vi "config.vi"(8 "error in (no error)":errorcluster, 10 "Configuration":T2={"Config Dir"=path "/home/ttsai/Documents/stash/ts_tcs_ofc/configData", "Config File Name"="optiPSSN_x00.ctrl", "Inst Name"=enum."lsst", "State 0 File Name"="state0inDof.txt", "Weighting File Name"="imgQualWgt.txt", "PSSN Alpha File Name"="pssn_alpha.txt", "Authority Files"={"Rigid Body Stroke File"="rbStroke.txt", "M1M3 Subsystem"={"Mirror"="M1M3", "Actuatro Force File"="M1M3_1um_156_force.DAT"}, "M2 Subsystem"={"Mirror"="M2", "Actuatro Force File"="M2_1um_force.DAT"}, "Num of Bending Mode"=20}}, 11 "OptCtrl in":refnum<class "OptCtrl.lvclass">) -> (0 "error out":errorcluster, 3 "OptCtrl out":refnum<class "OptCtrl.lvclass">)   [LabVIEW 2016, in "OptCtrl.lvclass"]
doc: "Do the configuration of optimal comtrol (OC)."
uses:
  OptCtrl.lvclass
  StrictDef/InstName.ctl
  OptCtrl.lvclass/OptCtrl.ctl
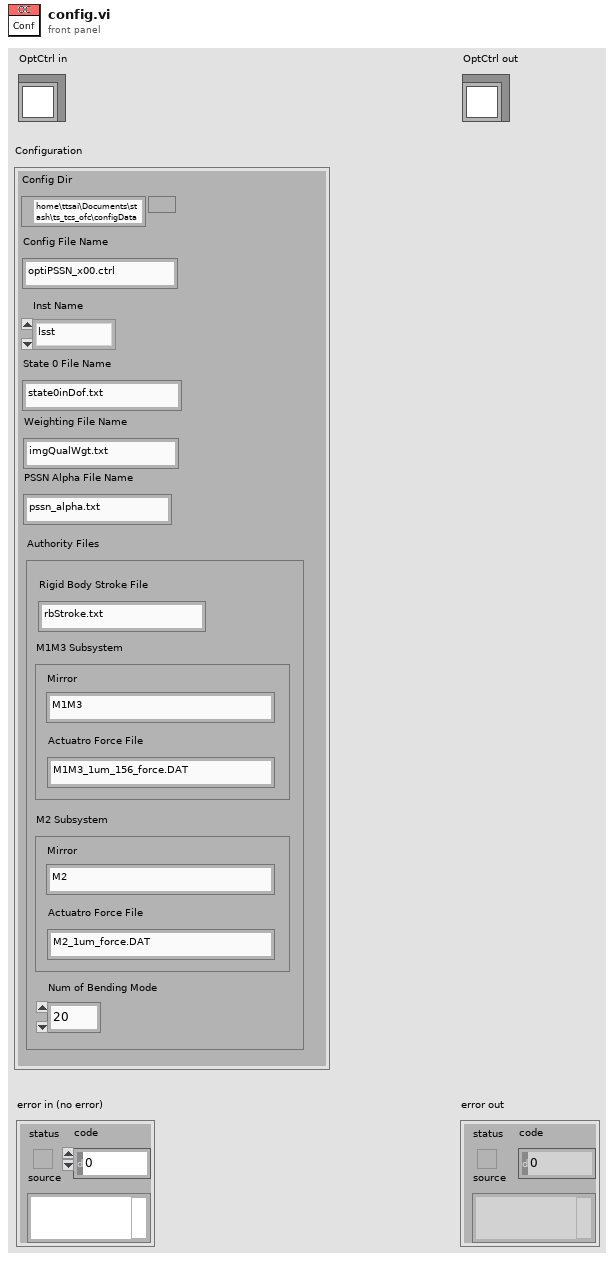
[diagram p1: front panel]
types:
  T1 = typedef "InstName.ctl" = enum16{"lsst", "comcam"}
  T2 = cluster{"Config Dir":path, "Config File Name":string, "Inst Name":T1, "State 0 File Name":string, "Weighting File Name":string, "PSSN Alpha File Name":string, "Authority Files":cluster{"Rigid Body Stroke File":string, "M1M3 Subsystem":cluster{"Mirror":string, "Actuatro Force File":string}, "M2 Subsystem":cluster{"Mirror":string, "Actuatro Force File":string}, "Num of Bending Mode":i32}}
  T3 = cluster{"Rigid Body Stroke File":string, "M1M3 Subsystem":cluster{"Mirror":string, "Actuatro Force File":string}, "M2 Subsystem":cluster{"Mirror":string, "Actuatro Force File":string}, "Num of Bending Mode":i32}
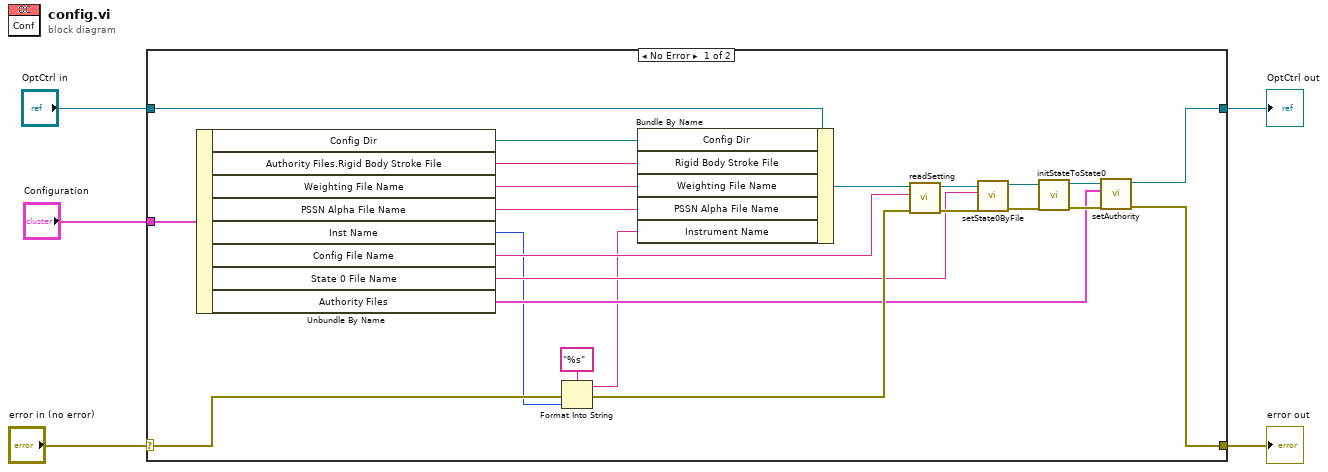
[diagram p0: block diagram]
diagram:
  n1 = case shown="No Error" "error in (no error)" {
    selector: "error in (no error)" -> [w24 w30]
    tunnel: [w15 w30] -> w4
    tunnel: [w16 w29] -> w2
    tunnel: "OptCtrl in" -> [w27 w29]
    tunnel: "Configuration" -> [w28 _]
    frame No Error {
      n2 = Unbundle By Name(w28) -> ("Config Dir"=w14:path, "Authority Files.Rigid Body Stroke File"=w13:string, "Weighting File Name"=w7:string, "PSSN Alpha File Name"=w6:string, "Inst Name"=w9:T1, "Config File Name"=w12:string, "State 0 File Name"=w11:string, "Authority Files"=w10:T3)
      n3 = Format Into String(format string="%s", error in=w24, w9) -> (resulting string=w8:string, error out=w23:errorcluster)  [unwired: 1 in]
      n4 = Bundle By Name(cluster=w27, "Config Dir"=w14, "Rigid Body Stroke File"=w13, "Weighting File Name"=w7, "PSSN Alpha File Name"=w6, "Instrument Name"=w8) -> (w26:refnum<class "OptCtrl.lvclass">)
      n5 = call "readSetting.vi"("error in (no error)"=w23, "Config File Name"=w12, "OptCtrl in"=w26) -> ("error out"=w21:errorcluster, "OptCtrl out"=w22:refnum<class "OptCtrl.lvclass">)  [unwired: 7 in]
      n6 = call "setState0ByFile.vi"("error in (no error)"=w21, "State 0 File Name"=w11, "OptCtrl in"=w22) -> ("error out"=w19:errorcluster, "OptCtrl out"=w20:refnum<class "OptCtrl.lvclass">)  [unwired: 7 in]
      n7 = call "initStateToState0.vi"("error in (no error)"=w19, "OptCtrl in"=w20) -> ("error out"=w17:errorcluster, "OptCtrl out"=w18:refnum<class "OptCtrl.lvclass">)  [unwired: 8 in]
      n8 = call "setAuthority.vi"("error in (no error)"=w17, "Authority Files"=w10, "OptCtrl in"=w18) -> ("error out"=w15:errorcluster, "OptCtrl out"=w16:refnum<class "OptCtrl.lvclass">)  [unwired: 7 in]
    }
    frame Error {
    }
  }
  "error out" <- w4
  "OptCtrl out" <- w2
